vi "csv data to separated text files.vi"() -> ()   [LabVIEW 2020]
uses:
  <vilib>/Waveform/WDTFileIO.llb/Export Waveforms To Spreadsheet File (1D).vi
panel:
  in  "Path":path
  out "Array":string[](array[string])
  out "output array":string[][][](array[string])
  out "header":string[](array[string])
  out "size(s)":i32[](array[numeric])
  in  "file (use dialog) in":path
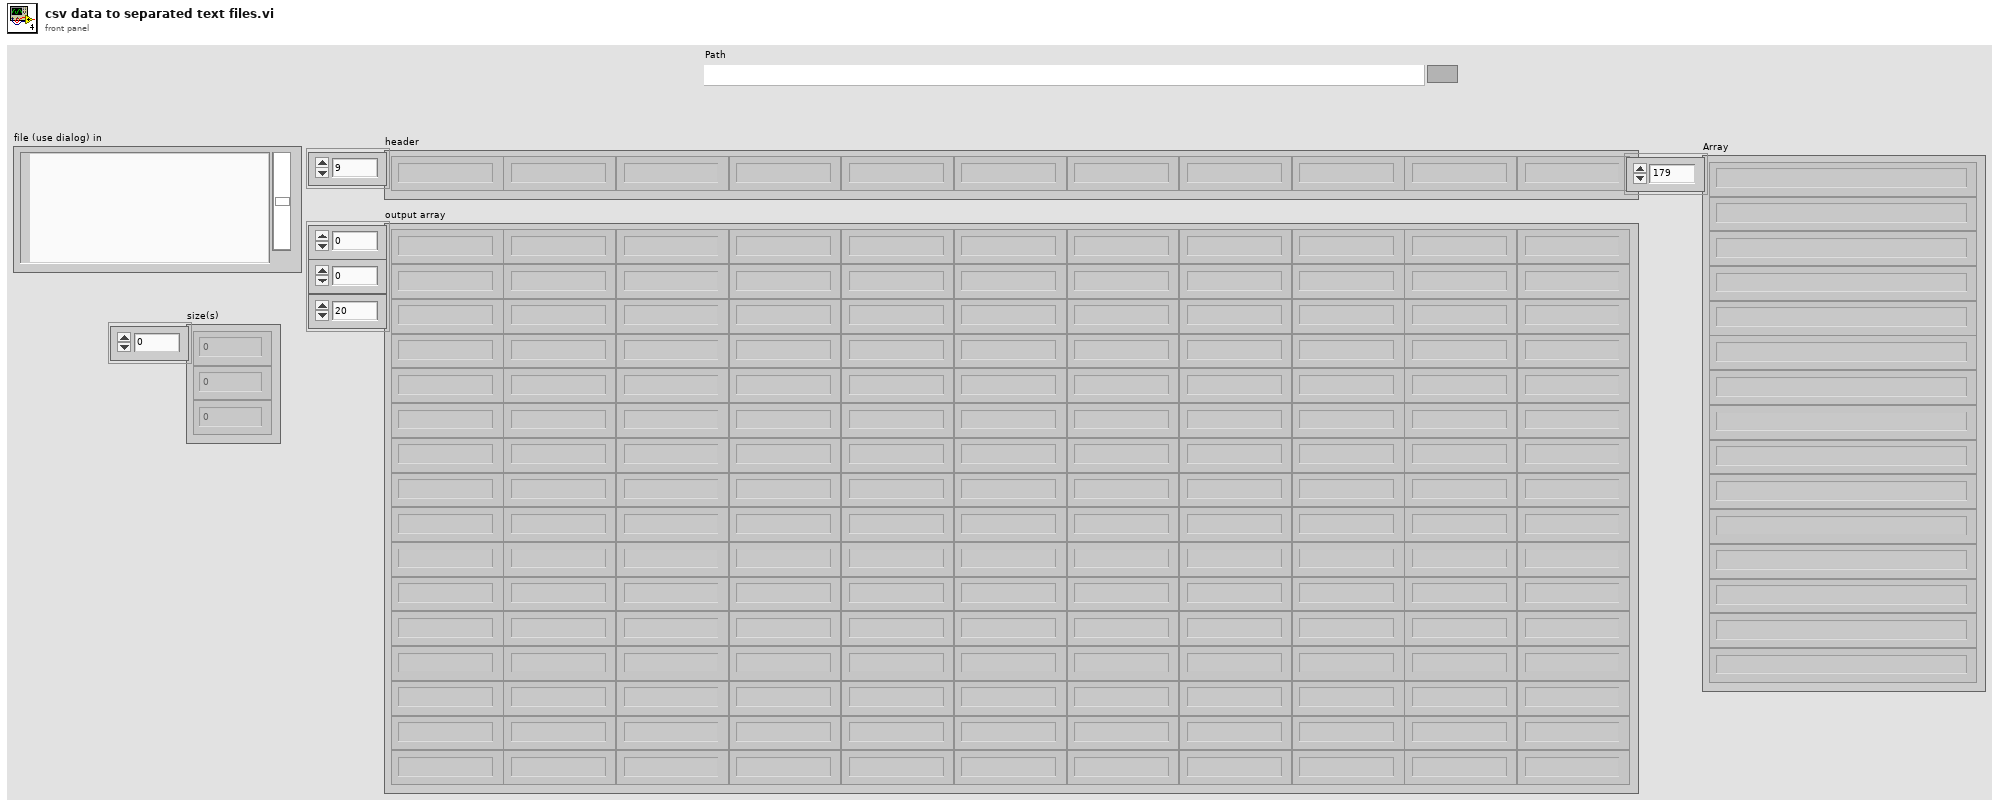
[diagram p1: front panel]
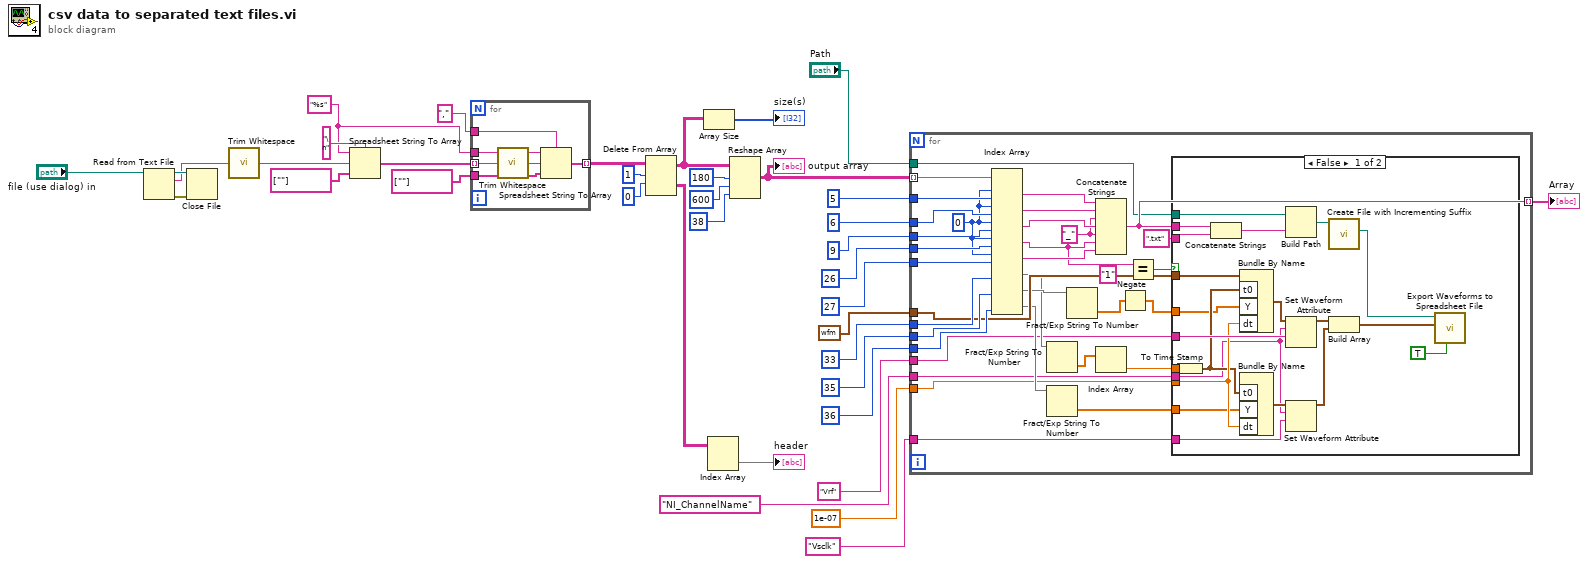
[diagram p0: block diagram]
diagram:
  w32 = "%s" ("format string")
  n1 = Read from Text File(file (use dialog)="file (use dialog) in") -> (refnum out=w37:refnum<file>, text=w21:string, error out=w36:errorcluster)  [unwired: 3 in, 1 out]
  n2 = Close File(refnum=w37, error in=w36) -> ()  [unwired: 2 out]
  n3 = call <vilib>:"Trim Whitespace.vi"("string"=w21) -> ("trimmed string"=w27:string)  [unwired: 1 in]
  n4 = Spreadsheet String To Array(delimiter (Tab)="\n", format string=w32, spreadsheet string=w27, array type (2D Dbl)=string[] [""]) -> (array=w31:string[])
  n5 = for {
    tunnel: "," ("delimiter (Tab)") -> [w43]
    tunnel: w32 -> [w42]
    tunnel: w31 -> [w39] mode=indexing
    tunnel: string[] [""] -> [w41]
    tunnel: [w40] -> w26 mode=indexing
    n6 = call <vilib>:"Trim Whitespace.vi"("string"=w39) -> ("trimmed string"=w38:string)  [unwired: 1 in]
    n7 = Spreadsheet String To Array(delimiter (Tab)=w43, format string=w42, spreadsheet string=w38, array type (2D Dbl)=w41) -> (array=w40:string[])
  }
  n8 = Delete From Array(array=w26, length=1, index (row)=0) -> (deleted portion=w23:string[][], array with subset deleted=w20:string[][])  [unwired: 1 in]
  n9 = Array Size(array=w20) -> (size(s)=→"size(s)":i32[])
  n10 = Index Array(array=w23) -> (element=→"header":string[])  [unwired: 2 in]
  n11 = Reshape Array(w20, 180 ("dimension size"), 600 ("dimension size"), 38 ("dimension size")) -> (w16:string[][][])
  "output array" <- w16
  n12 = for {
    tunnel: w16 -> [w77] mode=indexing
    tunnel: 5 ("dimension size") -> [w76]
    tunnel: 6 ("dimension size") -> [w75]
    tunnel: 9 ("dimension size") -> [w74]
    tunnel: 26 ("dimension size") -> [w73]
    tunnel: 27 ("dimension size") -> [w72]
    tunnel: 33 ("dimension size") -> [w71]
    tunnel: 35 ("dimension size") -> [w70]
    tunnel: 36 ("dimension size") -> [w69]
    tunnel: [w52] -> w7 mode=indexing
    tunnel: waveform(dbl) {"t0"=timestamp(0 s since 1904-01-01), "dt"=1.0, "Y"=[]} ("waveform") -> [w62]
    tunnel: 1e-07 ("dt") -> [w55]
    tunnel: "NI_ChannelName" ("name") -> [w54]
    tunnel: "Vrf" ("name") -> [w56]
    tunnel: "Vsclk" ("name") -> [w53]
    tunnel: "Path" -> [w50]
    w64 = "_" ("string")
    w66 = 0 ("disabled index (row)")
    n13 = Index Array(array=w77, index (row) #1=w66, index (col) #1=w76, index (row) #2=w66, index (col) #2=w75, index (row) #3=w66, index (col) #3=w74, index (row) #4=w66, index (col) #4=w73, index (row) #5=w66, index (col) #5=w72, index (col) #6=w71, index (col) #7=w70, index (col) #8=w69) -> (element #1=w68:string, element #2=w67:string, element #3=w65:string, element #4=w46:string, element #5=w63:string, element #6=w59:string[], element #7=w60:string[], element #8=w61:string[])  [unwired: 3 in]
    n14 = Fract/Exp String To Number(string=w59) -> (number=w58:dbl[])  [unwired: 3 in, 1 out]
    n15 = Fract/Exp String To Number(string=w61) -> (number=w49:dbl[])  [unwired: 3 in, 1 out]
    n16 = Fract/Exp String To Number(string=w60) -> (number=w48:dbl[])  [unwired: 3 in, 1 out]
    n17 = Concatenate Strings(w68, w67, w64, w65, w64, w46, w63) -> (w52:string)
    n18 = Index Array(array=w58) -> (element=w57:dbl)  [unwired: 1 in]
    n19 = Negate(x=w48) -> (-x=w47:dbl[])
    n20 = Equal?(x=w46, y="1") -> (x = y?=w44:bool)
    n21 = case shown="False" w44 {
      tunnel: w62 -> [w98 _]
      tunnel: w57 -> [w96 _]
      tunnel: w56 -> [w95 _]
      tunnel: w55 -> [w93 _]
      tunnel: w54 -> [w91 _]
      tunnel: w53 -> [w90 _]
      tunnel: w52 -> [w86 _]
      tunnel: ".txt" ("string") -> [w85 _]
      tunnel: w50 -> [w83 _]
      tunnel: w49 -> [w82 _]
      tunnel: w47 -> [w79 _]
      frame False {
        n22 = To Time Stamp(1:w96) -> (0:w92:timestamp)
        n23 = Concatenate Strings(w86, w85) -> (w84:string)
        n24 = Bundle By Name(cluster=w98, "t0"=w92, "Y"=w79, "dt"=w93) -> (w97:waveform(dbl))
        n25 = Bundle By Name("t0"=w92, "Y"=w82, "dt"=w93) -> (w94:waveform(dbl))  [unwired: 1 in]
        n26 = Build Path(base path=w83, name or relative path=w84) -> (appended path=w81:path)
        n27 = Set Waveform Attribute(5:w95, 6:w91, 7:w97) -> (3:w89:waveform(dbl))  [unwired: 1 in, 2 out]
        n28 = Set Waveform Attribute(5:w90, 6:w91, 7:w94) -> (3:w88:waveform(dbl))  [unwired: 1 in, 2 out]
        n29 = call <vilib>:"Create File with Incrementing Suffix.vi"("file path"=w81) -> ("actual path"=w80:path)  [unwired: 8 in, 2 out]
        n30 = Build Array(w89, w88) -> (w87:waveform(dbl)[])
        n31 = call-poly <vilib>:"Export Waveforms to Spreadsheet File.vi"("append to file? (new file:F)"=TRUE, "waveforms"=w87, "file path (dialog if empty)"=w80) -> ()  [unwired: 7 in, 2 out]
      }
      frame True {
      }
    }
  }
  "Array" <- w7
